vi "Validate Semaphore Size.vi"(4 "error in (no error)":errorcluster, 7 "size (1)":i32) -> (0 "error out":errorcluster)   [LabVIEW 2020]
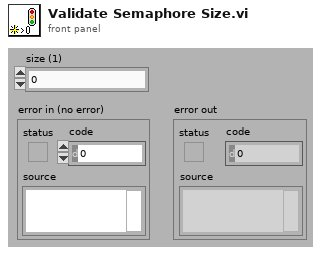
[diagram p1: front panel]
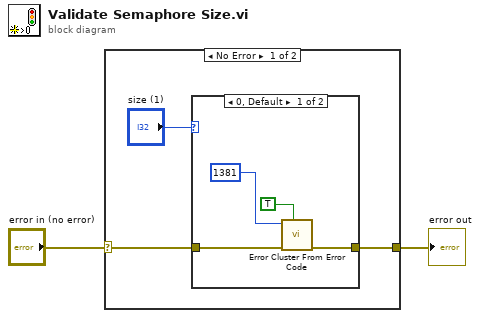
[diagram p0: block diagram]
diagram:
  n1 = case shown="No Error" "error in (no error)" {
    selector: "error in (no error)" -> [w3 w11]
    tunnel: [w4 w11] -> w1
    frame No Error {
      n2 = case shown="0, Default" "size (1)" {
        tunnel: [w7 w10] -> w4
        tunnel: w3 -> [w8 w10]
        frame 0, Default {
          n3 = call "Error Cluster From Error Code.vi"("show call chain? (False)"=TRUE, "error in (no error)"=w8, "error code (0)"=1381 ("code")) -> ("error out"=w7:errorcluster)  [unwired: 6 out]
        }
        frame 1.. {
        }
      }
    }
    frame Error {
    }
  }
  "error out" <- w1
